vi "BoolCmd_Send.vi"(7 "Command Name":string) -> (0 "error out":errorcluster)   [LabVIEW 2019, in "Trajectory_Library.lvlib"]
uses:
  Trajectory_Library.lvlib
  BoolCmd_ObtainQueue.vi
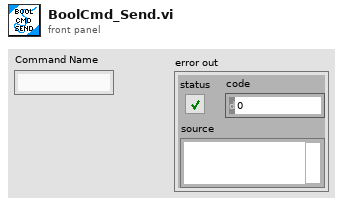
[diagram p1: front panel]
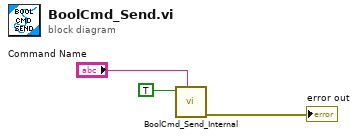
[diagram p0: block diagram]
diagram:
  n1 = call "BoolCmd_Send_Internal.vi"("Command Name"="Command Name", "Value"=TRUE) -> ("error out"=→"error out":errorcluster)  [unwired: 9 in]
